vi "dequeue_commands.vi"(8 "error in (no error)":errorcluster caption="错误输入（无错误）", 11 "MotorSystem输入":refnum<class "MotorSystem.lvclass">) -> (0 "error out":errorcluster caption="错误输出", 2 "command cluster":cluster{"cmd":T1, "cmd data":variant}, 3 "MotorSystem输出":refnum<class "MotorSystem.lvclass">)   [LabVIEW 2016, in "MotionControl_UFO_3DOF.lvlib" / "MotorSystem.lvclass"]
uses:
  <userlib>/MotionControl_UFO_3DOF/MotorSystem/MotorSystem.lvclass
  <userlib>/MotionControl_UFO_3DOF/MotorSystem/cmd_system.ctl
  <userlib>/MotionControl_UFO_3DOF/MotorSystem/MotorSystem.lvclass/MotorSystem.ctl
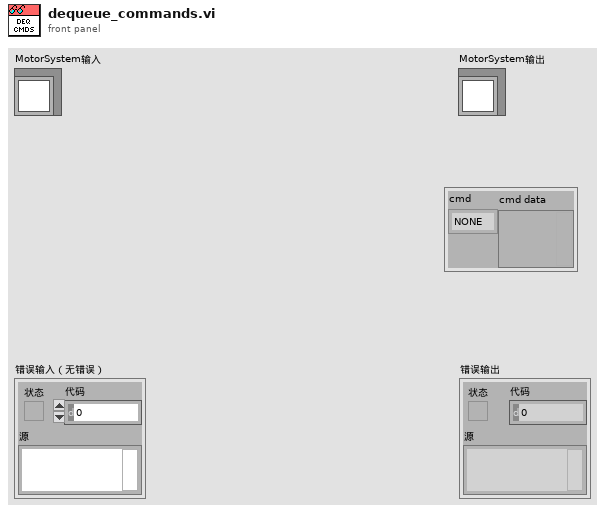
[diagram p1: front panel]
types:
  T1 = typedef "MotionControl_UFO_3DOF.lvlib/MotorSystem.lvclass/cmd_system.ctl" = enum16{"NONE", "MOVE_SYSTEM", "WAIT_UNTIL_MOVE_DONE", "EXIT", "WAIT_UNTIL_SELECTED_MOVE_DONE", "WAIT_A_TIME"}
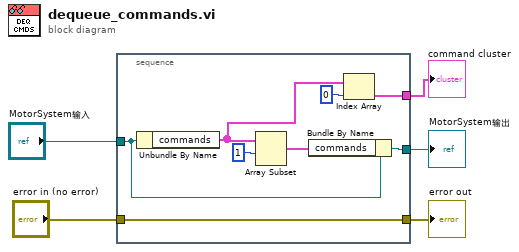
[diagram p0: block diagram]
diagram:
  n1 = stacked-sequence {
    tunnel: [w6] -> w5
    tunnel: [w7] -> w3
    tunnel: "MotorSystem输入" -> [w8]
    tunnel: [w10] -> w2
    tunnel: "error in (no error)" -> [w6]
    frame #0 {
      n2 = Unbundle By Name(w8) -> ("commands"=w12:cluster{"cmd":T1, "cmd data":variant}[])
      n3 = Array Subset(array=w12, index=1 ("索引")) -> (w9:cluster{"cmd":T1, "cmd data":variant}[])  [unwired: 1 in]
      n4 = Bundle By Name(cluster=w8, "commands"=w9) -> (w7:refnum<class "MotorSystem.lvclass">)
      n5 = Index Array(array=w12, index=0 ("索引")) -> (element=w10:cluster{"cmd":T1, "cmd data":variant})
    }
  }
  "error out" <- w5
  "MotorSystem输出" <- w3
  "command cluster" <- w2
